vi "PigeonSetStatusRates.vi"(9 "Pigeon IMU Set Status Rates":T1={"General (ms)"=20, "Six Deg YPR (ms)"=200, "Sensor Fushion (ms)"=50, "General Compass (ms)"=200, "Gyro Accum (ms)"=100, "General Accel (ms)"=50, "Biased Accel (ms)"=200, "Biased Mag (ms)"=200, "Gyro (ms)"=100, "Raw Mag (ms)"=200, "Six Deg Quat (ms)"=200}, 11 "PigeonIMU DevRef In":T2={"DeviceStatus"={"status"=FALSE, "code"=0, "source"=""}, "Device Number"=0, "Type"=352321536, "Device ID"=0, "Handle"=0, "UsageFrame"=0, "Library Path"=path ""} {"Type" items=["CAN"=352321536, "TalonSRX"=33554432]}) -> (3 "PigeonIMU DevRef Out":T2={"DeviceStatus"={"status"=FALSE, "code"=0, "source"=""}, "Device Number"=0, "Type"=352321536, "Device ID"=0, "Handle"=0, "UsageFrame"=0, "Library Path"=path ""} {"Type" items=["CAN"=352321536, "TalonSRX"=33554432]})   [LabVIEW 2018]
uses:
  <vilib>/Rock Robotics/WPI/ThirdParty/Phoenix-LabVIEW/Pigeon IMU/CTRE_PigeonIMU_DeviceRef.ctl
  <vilib>/Rock Robotics/WPI/ThirdParty/Phoenix-LabVIEW/Pigeon IMU/CTRE_PigeonIMU_ConnectionType.ctl
  <vilib>/Rock Robotics/WPI/ThirdParty/Phoenix-LabVIEW/Pigeon IMU/CTRE_PigeonIMU_StatusFrameRate.ctl
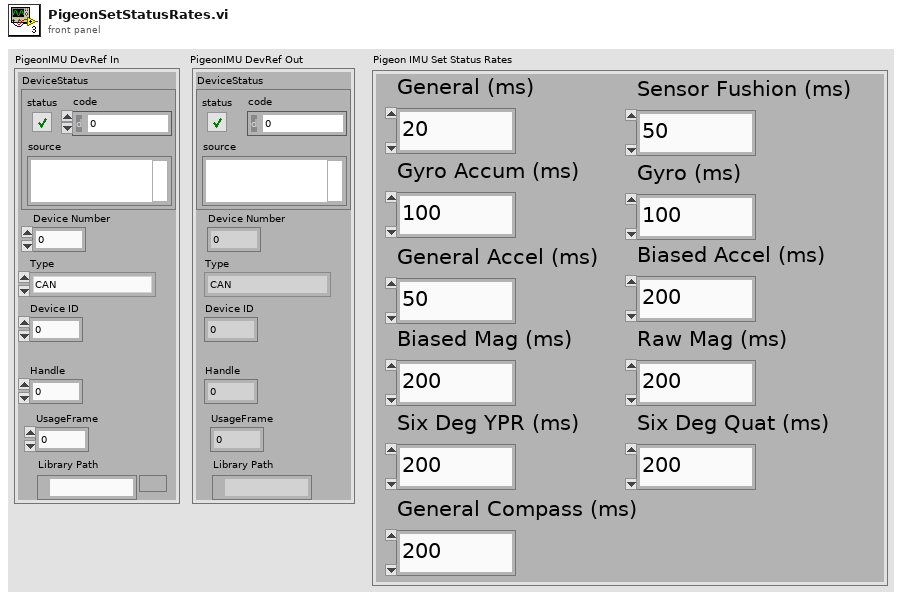
[diagram p1: front panel]
types:
  T1 = cluster{"General (ms)":i16, "Six Deg YPR (ms)":i16, "Sensor Fushion (ms)":i16, "General Compass (ms)":i16, "Gyro Accum (ms)":i16, "General Accel (ms)":i16, "Biased Accel (ms)":i16, "Biased Mag (ms)":i16, "Gyro (ms)":i16, "Raw Mag (ms)":i16, "Six Deg Quat (ms)":i16}
  T2 = typedef "CTRE_PigeonIMU_DeviceRef.ctl" = cluster{"DeviceStatus":errorcluster, "Device Number":u8, "Type":T3, "Device ID":u32, "Handle":u64, "UsageFrame":u32, "Library Path":path}
  T3 = typedef "CTRE_PigeonIMU_ConnectionType.ctl" = u32
  T4 = typedef "CTRE_PigeonIMU_StatusFrameRate.ctl" = u32
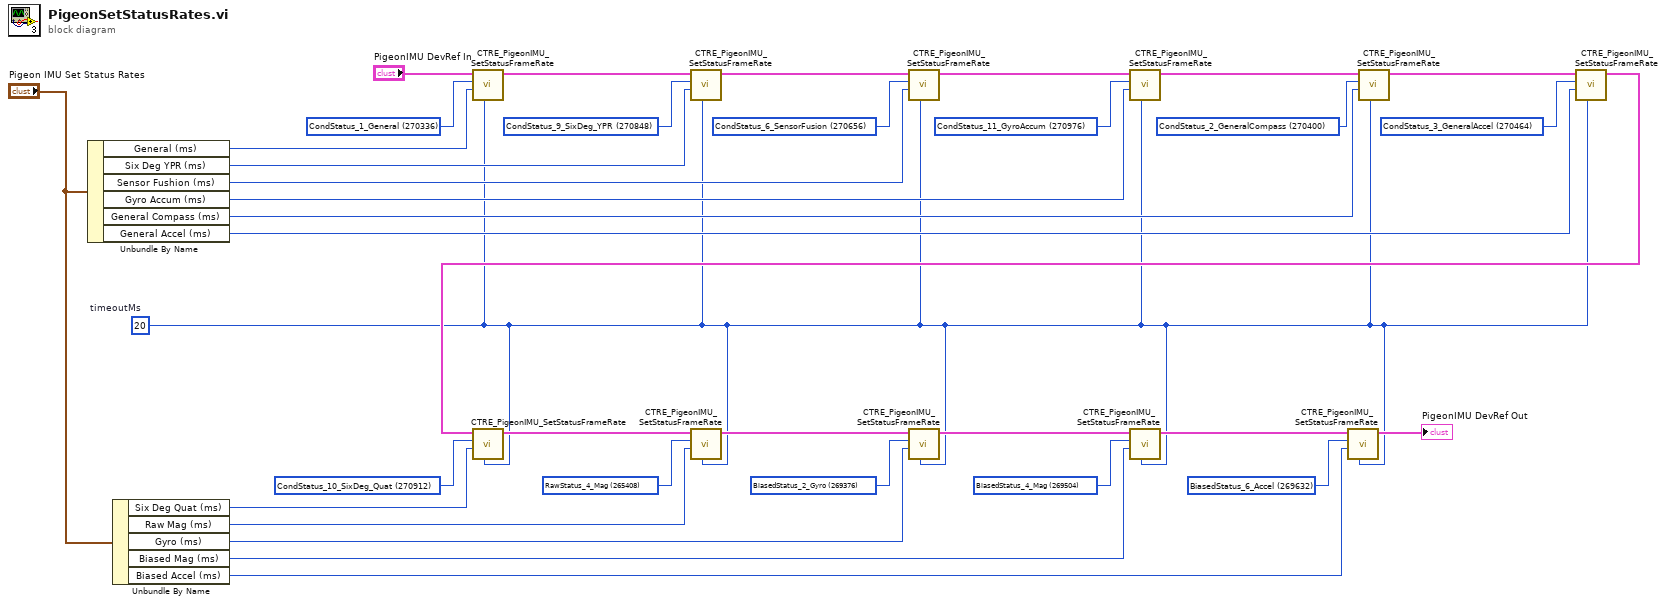
[diagram p0: block diagram]
diagram:
  w1 = u32 20  # timeoutMs
  w29 = T4 269632 items=["CondStatus_1_General"=270336, "CondStatus_9_SixDeg_YPR"=270848, "CondStatus_6_SensorFusion"=270656, "CondStatus_11_GyroAccum"=270976, "CondStatus_2_GeneralCompass"=270400, "CondStatus_3_GeneralAccel"=270464, "CondStatus_10_SixDeg_Quat"=270912, "RawStatus_4_Mag"=265408, "BiasedStatus_2_Gyro"=269376, "BiasedStatus_4_Mag"=269504, "BiasedStatus_6_Accel"=269632] ("StatusFrame")
  w30 = T4 269504 items=["CondStatus_1_General"=270336, "CondStatus_9_SixDeg_YPR"=270848, "CondStatus_6_SensorFusion"=270656, "CondStatus_11_GyroAccum"=270976, "CondStatus_2_GeneralCompass"=270400, "CondStatus_3_GeneralAccel"=270464, "CondStatus_10_SixDeg_Quat"=270912, "RawStatus_4_Mag"=265408, "BiasedStatus_2_Gyro"=269376, "BiasedStatus_4_Mag"=269504, "BiasedStatus_6_Accel"=269632] ("StatusFrame")
  w28 = T4 269376 items=["CondStatus_1_General"=270336, "CondStatus_9_SixDeg_YPR"=270848, "CondStatus_6_SensorFusion"=270656, "CondStatus_11_GyroAccum"=270976, "CondStatus_2_GeneralCompass"=270400, "CondStatus_3_GeneralAccel"=270464, "CondStatus_10_SixDeg_Quat"=270912, "RawStatus_4_Mag"=265408, "BiasedStatus_2_Gyro"=269376, "BiasedStatus_4_Mag"=269504, "BiasedStatus_6_Accel"=269632] ("StatusFrame")
  w27 = T4 265408 items=["CondStatus_1_General"=270336, "CondStatus_9_SixDeg_YPR"=270848, "CondStatus_6_SensorFusion"=270656, "CondStatus_11_GyroAccum"=270976, "CondStatus_2_GeneralCompass"=270400, "CondStatus_3_GeneralAccel"=270464, "CondStatus_10_SixDeg_Quat"=270912, "RawStatus_4_Mag"=265408, "BiasedStatus_2_Gyro"=269376, "BiasedStatus_4_Mag"=269504, "BiasedStatus_6_Accel"=269632] ("StatusFrame")
  w26 = T4 270912 items=["CondStatus_1_General"=270336, "CondStatus_9_SixDeg_YPR"=270848, "CondStatus_6_SensorFusion"=270656, "CondStatus_11_GyroAccum"=270976, "CondStatus_2_GeneralCompass"=270400, "CondStatus_3_GeneralAccel"=270464, "CondStatus_10_SixDeg_Quat"=270912, "RawStatus_4_Mag"=265408, "BiasedStatus_2_Gyro"=269376, "BiasedStatus_4_Mag"=269504, "BiasedStatus_6_Accel"=269632] ("StatusFrame")
  w31 = T4 270464 items=["CondStatus_1_General"=270336, "CondStatus_9_SixDeg_YPR"=270848, "CondStatus_6_SensorFusion"=270656, "CondStatus_11_GyroAccum"=270976, "CondStatus_2_GeneralCompass"=270400, "CondStatus_3_GeneralAccel"=270464, "CondStatus_10_SixDeg_Quat"=270912, "RawStatus_4_Mag"=265408, "BiasedStatus_2_Gyro"=269376, "BiasedStatus_4_Mag"=269504, "BiasedStatus_6_Accel"=269632] ("StatusFrame")
  w33 = T4 270400 items=["CondStatus_1_General"=270336, "CondStatus_9_SixDeg_YPR"=270848, "CondStatus_6_SensorFusion"=270656, "CondStatus_11_GyroAccum"=270976, "CondStatus_2_GeneralCompass"=270400, "CondStatus_3_GeneralAccel"=270464, "CondStatus_10_SixDeg_Quat"=270912, "RawStatus_4_Mag"=265408, "BiasedStatus_2_Gyro"=269376, "BiasedStatus_4_Mag"=269504, "BiasedStatus_6_Accel"=269632] ("StatusFrame")
  w32 = T4 270976 items=["CondStatus_1_General"=270336, "CondStatus_9_SixDeg_YPR"=270848, "CondStatus_6_SensorFusion"=270656, "CondStatus_11_GyroAccum"=270976, "CondStatus_2_GeneralCompass"=270400, "CondStatus_3_GeneralAccel"=270464, "CondStatus_10_SixDeg_Quat"=270912, "RawStatus_4_Mag"=265408, "BiasedStatus_2_Gyro"=269376, "BiasedStatus_4_Mag"=269504, "BiasedStatus_6_Accel"=269632] ("StatusFrame")
  w34 = T4 270656 items=["CondStatus_1_General"=270336, "CondStatus_9_SixDeg_YPR"=270848, "CondStatus_6_SensorFusion"=270656, "CondStatus_11_GyroAccum"=270976, "CondStatus_2_GeneralCompass"=270400, "CondStatus_3_GeneralAccel"=270464, "CondStatus_10_SixDeg_Quat"=270912, "RawStatus_4_Mag"=265408, "BiasedStatus_2_Gyro"=269376, "BiasedStatus_4_Mag"=269504, "BiasedStatus_6_Accel"=269632] ("StatusFrame")
  w35 = T4 270848 items=["CondStatus_1_General"=270336, "CondStatus_9_SixDeg_YPR"=270848, "CondStatus_6_SensorFusion"=270656, "CondStatus_11_GyroAccum"=270976, "CondStatus_2_GeneralCompass"=270400, "CondStatus_3_GeneralAccel"=270464, "CondStatus_10_SixDeg_Quat"=270912, "RawStatus_4_Mag"=265408, "BiasedStatus_2_Gyro"=269376, "BiasedStatus_4_Mag"=269504, "BiasedStatus_6_Accel"=269632] ("StatusFrame")
  w36 = T4 270336 items=["CondStatus_1_General"=270336, "CondStatus_9_SixDeg_YPR"=270848, "CondStatus_6_SensorFusion"=270656, "CondStatus_11_GyroAccum"=270976, "CondStatus_2_GeneralCompass"=270400, "CondStatus_3_GeneralAccel"=270464, "CondStatus_10_SixDeg_Quat"=270912, "RawStatus_4_Mag"=265408, "BiasedStatus_2_Gyro"=269376, "BiasedStatus_4_Mag"=269504, "BiasedStatus_6_Accel"=269632] ("StatusFrame")
  n1 = Unbundle By Name("Pigeon IMU Set Status Rates") -> ("General (ms)"=w13:i16, "Six Deg YPR (ms)"=w12:i16, "Sensor Fushion (ms)"=w11:i16, "Gyro Accum (ms)"=w10:i16, "General Compass (ms)"=w9:i16, "General Accel (ms)"=w8:i16)
  n2 = Unbundle By Name("Pigeon IMU Set Status Rates") -> ("Six Deg Quat (ms)"=w7:i16, "Raw Mag (ms)"=w6:i16, "Gyro (ms)"=w5:i16, "Biased Mag (ms)"=w4:i16, "Biased Accel (ms)"=w3:i16)
  n3 = call <vilib>:"CTRE_PigeonIMU_SetStatusFrameRate.vi"("timeoutMs"=w1, "Period (ms)"=w13, "StatusFrame"=w36, "PigeonIMUDevRef"="PigeonIMU DevRef In") -> ("PigeonIMUDevRef"=w20:T2)  [unwired: 6 in, 1 out]
  n4 = call <vilib>:"CTRE_PigeonIMU_SetStatusFrameRate.vi"("timeoutMs"=w1, "Period (ms)"=w12, "StatusFrame"=w35, "PigeonIMUDevRef"=w20) -> ("PigeonIMUDevRef"=w21:T2)  [unwired: 6 in, 1 out]
  n5 = call <vilib>:"CTRE_PigeonIMU_SetStatusFrameRate.vi"("timeoutMs"=w1, "Period (ms)"=w11, "StatusFrame"=w34, "PigeonIMUDevRef"=w21) -> ("PigeonIMUDevRef"=w22:T2)  [unwired: 6 in, 1 out]
  n6 = call <vilib>:"CTRE_PigeonIMU_SetStatusFrameRate.vi"("timeoutMs"=w1, "Period (ms)"=w10, "StatusFrame"=w32, "PigeonIMUDevRef"=w22) -> ("PigeonIMUDevRef"=w23:T2)  [unwired: 6 in, 1 out]
  n7 = call <vilib>:"CTRE_PigeonIMU_SetStatusFrameRate.vi"("timeoutMs"=w1, "Period (ms)"=w9, "StatusFrame"=w33, "PigeonIMUDevRef"=w23) -> ("PigeonIMUDevRef"=w24:T2)  [unwired: 6 in, 1 out]
  n8 = call <vilib>:"CTRE_PigeonIMU_SetStatusFrameRate.vi"("timeoutMs"=w1, "Period (ms)"=w8, "StatusFrame"=w31, "PigeonIMUDevRef"=w24) -> ("PigeonIMUDevRef"=w25:T2)  [unwired: 6 in, 1 out]
  n9 = call <vilib>:"CTRE_PigeonIMU_SetStatusFrameRate.vi"("timeoutMs"=w1, "Period (ms)"=w7, "StatusFrame"=w26, "PigeonIMUDevRef"=w25) -> ("PigeonIMUDevRef"=w19:T2)  [unwired: 6 in, 1 out]
  n10 = call <vilib>:"CTRE_PigeonIMU_SetStatusFrameRate.vi"("timeoutMs"=w1, "Period (ms)"=w6, "StatusFrame"=w27, "PigeonIMUDevRef"=w19) -> ("PigeonIMUDevRef"=w18:T2)  [unwired: 6 in, 1 out]
  n11 = call <vilib>:"CTRE_PigeonIMU_SetStatusFrameRate.vi"("timeoutMs"=w1, "Period (ms)"=w5, "StatusFrame"=w28, "PigeonIMUDevRef"=w18) -> ("PigeonIMUDevRef"=w17:T2)  [unwired: 6 in, 1 out]
  n12 = call <vilib>:"CTRE_PigeonIMU_SetStatusFrameRate.vi"("timeoutMs"=w1, "Period (ms)"=w4, "StatusFrame"=w30, "PigeonIMUDevRef"=w17) -> ("PigeonIMUDevRef"=w16:T2)  [unwired: 6 in, 1 out]
  n13 = call <vilib>:"CTRE_PigeonIMU_SetStatusFrameRate.vi"("timeoutMs"=w1, "Period (ms)"=w3, "StatusFrame"=w29, "PigeonIMUDevRef"=w16) -> ("PigeonIMUDevRef"=→"PigeonIMU DevRef Out":T2)  [unwired: 6 in, 1 out]
